vi "Dual_input_latch.vi"(9 "Reset on\nFirst Call?(T)":bool=TRUE, 10 "Reset":bool, 11 "Set":bool) -> (3 "Latched?":bool)   [LabVIEW 2012]
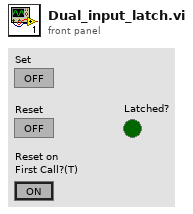
[diagram p1: front panel]
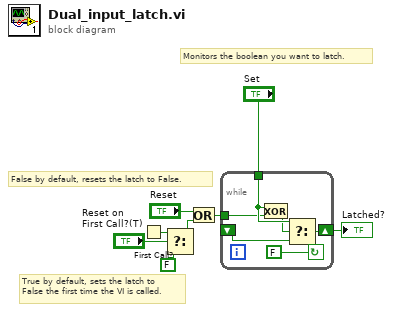
[diagram p0: block diagram]
diagram:
  # "Monitors the boolean you want to latch."
  # "False by default, resets the latch to False."
  # "True by default, sets the latch to\nFalse the first time the VI is called."
  n1 = First Call?() -> (First Call?: T/F=w3:bool)
  n2 = Select(t=w3, s="Reset on\nFirst Call?(T)", f=FALSE) -> (s? t:f=w4:bool)
  n3 = Or(x="Reset", y=w4) -> (x .or. y?=w6:bool)
  n4 = while {
    tunnel: "Set" -> [w14]
    shift-right: [w12] -> w7
    shift-left: _ -> [w11]
    tunnel: w6 -> [w9]
    stop <- FALSE continue-if-true
    n5 = Exclusive Or(1:w9, 2:w14) -> (0:w13:bool)
    n6 = Select(t=w14, s=w13, f=w11) -> (s? t:f=w12:bool)
  }
  "Latched?" <- w7
